vi "TCU Settings Dialog.vi"(8 "error in (no error)":errorcluster, 10 "Message Queues":T11, 11 "TCU Module State Cluster In":T1={"TCU Module Config"={"GUID"="", "Drop Coords"={"Horizontal"=0, "Vertical"=0}, "Process Name"="", "User name"="", "Queue Name"="", "Settings"={"Cycle Period"=500.0, "Setpoint Entry"=0.0, "Output Device"=enum."Default", "Huber Ministat 230 Settings"={"VISA resource name"="", "Simulated?"=TRUE}, "Lauda Settings"={"VISA resource name"="", "Simulated?"=FALSE, "Pump Power"=2}, "Julabo FP-50 Settings"={"VISA resource name"="", "Simulated?"=FALSE, "Pump Power"=2}, "Internal Control?"=FALSE, "Huber Unistat 410 Settings"={"VISA resource name"="", "Address"=0, "Simulated?"=FALSE}}, "Load Count"=0, "Power Level Changed"=FALSE}, "State"=enum."Idle", "Start Time"=timestamp(0 s since 1904-01-01), "Current Time"=timestamp(0 s since 1904-01-01), "First Iteration"=FALSE, "Data"={"TCU Temp"=0.0}, "Process Name"="", "TCU On?"=FALSE, "Power Level Changed"=FALSE} {"TCU Module Config"."Settings"."Huber Unistat 410 Settings"."Address" min=0 max=99 format="%02.0f"; "TCU Module Config"."Settings"."Julabo FP-50 Settings"."Pump Power" min=0 max=8 step=1; "TCU Module Config"."Settings"."Lauda Settings"."Pump Power" min=0 max=8 step=1}) -> (0 "error out":errorcluster, 1 "Cancelled?":bool=TRUE, 2 "UI Refresh Needed?":bool, 3 "TCU Module Config Out":T2={"GUID"="", "Drop Coords"={"Horizontal"=0, "Vertical"=0}, "Process Name"="", "User name"="", "Queue Name"="", "Settings"={"Cycle Period"=0.0, "Setpoint Entry"=0.0, "Output Device"=enum."Default", "Huber Ministat 230 Settings"={"VISA resource name"="", "Simulated?"=FALSE}, "Lauda Settings"={"VISA resource name"="", "Simulated?"=FALSE, "Pump Power"=2}, "Julabo FP-50 Settings"={"VISA resource name"="", "Simulated?"=FALSE, "Pump Power"=2}, "Internal Control?"=FALSE, "Huber Unistat 410 Settings"={"VISA resource name"="", "Address"=0, "Simulated?"=FALSE}}, "Load Count"=0, "Power Level Changed"=FALSE} {"Settings"."Huber Unistat 410 Settings"."Address" min=0 max=99 format="%02.0f"; "Settings"."Julabo FP-50 Settings"."Pump Power" min=0 max=8 step=1; "Settings"."Lauda Settings"."Pump Power" min=0 max=8 step=1})   [LabVIEW 2018, in "TCU Module.lvlib"]
doc: "Dialog for selecting user specified settings."
uses:
  TCU Module.lvlib
  Ismatec ISM 831C/Controls/Ismatech ISM831C Settings Cluster.ctl
  Masterflex 7550-30/Controls/Settings Cluster.ctl
  VICI M50/VICI Settings.ctl
  Measure Instrument/Output Devices.ctl
  Huber TCU/Huber Settings.ctl
  Julabo Type 1 TCU/Julabo Type 1 TCU Folder/Julabo FP-50 Settings.ctl
  Lauda Integral XT-150 TCU/Lauda Settings.ctl
  Huber Unistat 410 TCU/Huber Unistat 410 RS485 Settings.ctl
  All Message Queues.ctl
  support/Message Queue/Message Cluster.ctl
  TCU Module Config Cluster.ctl
  <vilib>/Utility/miscctls.llb/LVPoint32TypeDef.ctl
  TCU Module Settings Cluster.ctl
  TCU Module State Cluster.ctl
  Measure Instrument/State Enum.ctl
  support/Message Queue/Enqueue Message (Single).vi
  <vilib>/Utility/xml.llb/Write to XML File(string).vi
  Settings/Settings.lvlib
  support/Support Library.lvlib
  support/Message Queue/Message Queue.lvlib
  Huber TCU/Huber Ministat 230 TCU.lvlib
  Lauda Integral XT-150 TCU/Lauda TCU.lvlib
  Julabo Type 1 TCU/Julabo Type 1 TCU Folder/Julabo Type FP-50 TCU.lvlib
  Huber Unistat 410 TCU/Huber Unistat 410 TCU.lvlib
  Ismatec ISM 831C/Ismatec ISM 831C.lvlib
  Masterflex 7550-30/Masterflex 7550-30.lvlib
  Measure Instrument/Feed Module Engine.lvlib
panel:
  in  "Module Name":string
  in  "TCU Settings":T15={"TCU Configuration"={"Cycle Period"=500.0, "Ismatech"={"VISA resource name"="", "Simulated?"=FALSE, "Pump Number"=1.0, "Reverse?"=FALSE}, "Masterflex"={"VISA resource name"="", "Simulated?"=FALSE, "Pump Number"=1.0, "Reverse?"=FALSE}, "Setpoint Entry"=0.0, "VICI Settings"={"VISA resource name"="", "Simulated?"=FALSE, "Pump Number"=0.0, "Reverse?"=FALSE}, "Output Device"=enum."Default", "Huber Ministat 230 Settings"={"VISA resource name"="", "Simulated?"=FALSE}, "Julabo Type 1 Settings"={"VISA resource name"="", "Simulated?"=FALSE, "Pump Power"=2}, "Lauda Settings"={"VISA resource name"="", "Simulated?"=FALSE, "Pump Power"=2}, "Control"=enum."Internal", "Huber Unistat 410 Settings"={"VISA resource name"="", "Address"=0, "Simulated?"=FALSE}}, "Stop"=FALSE, "Start"=FALSE} {"TCU Configuration"."Huber Unistat 410 Settings"."Address" min=0 max=99 format="%02.0f"; "TCU Configuration"."Lauda Settings"."Pump Power" min=0 max=8 step=1; "TCU Configuration"."Julabo Type 1 Settings"."Pump Power" min=0 max=8 step=1; "TCU Configuration"."VICI Settings"."Pump Number" min=1.0 max=20.0 step=1.0; "TCU Configuration"."Ismatech"."Pump Number" min=1.0 max=20.0 step=1.0; "TCU Configuration"."Masterflex"."Pump Number" min=1.0 max=20.0 step=1.0}
  in  "Cancel Button":bool
  in  "OK Button":bool
  # "Non visible portion of dialog (needed for connector pane)."
  # "Output Instruments"
  # "Output Instruments"
  # "Output Instruments"
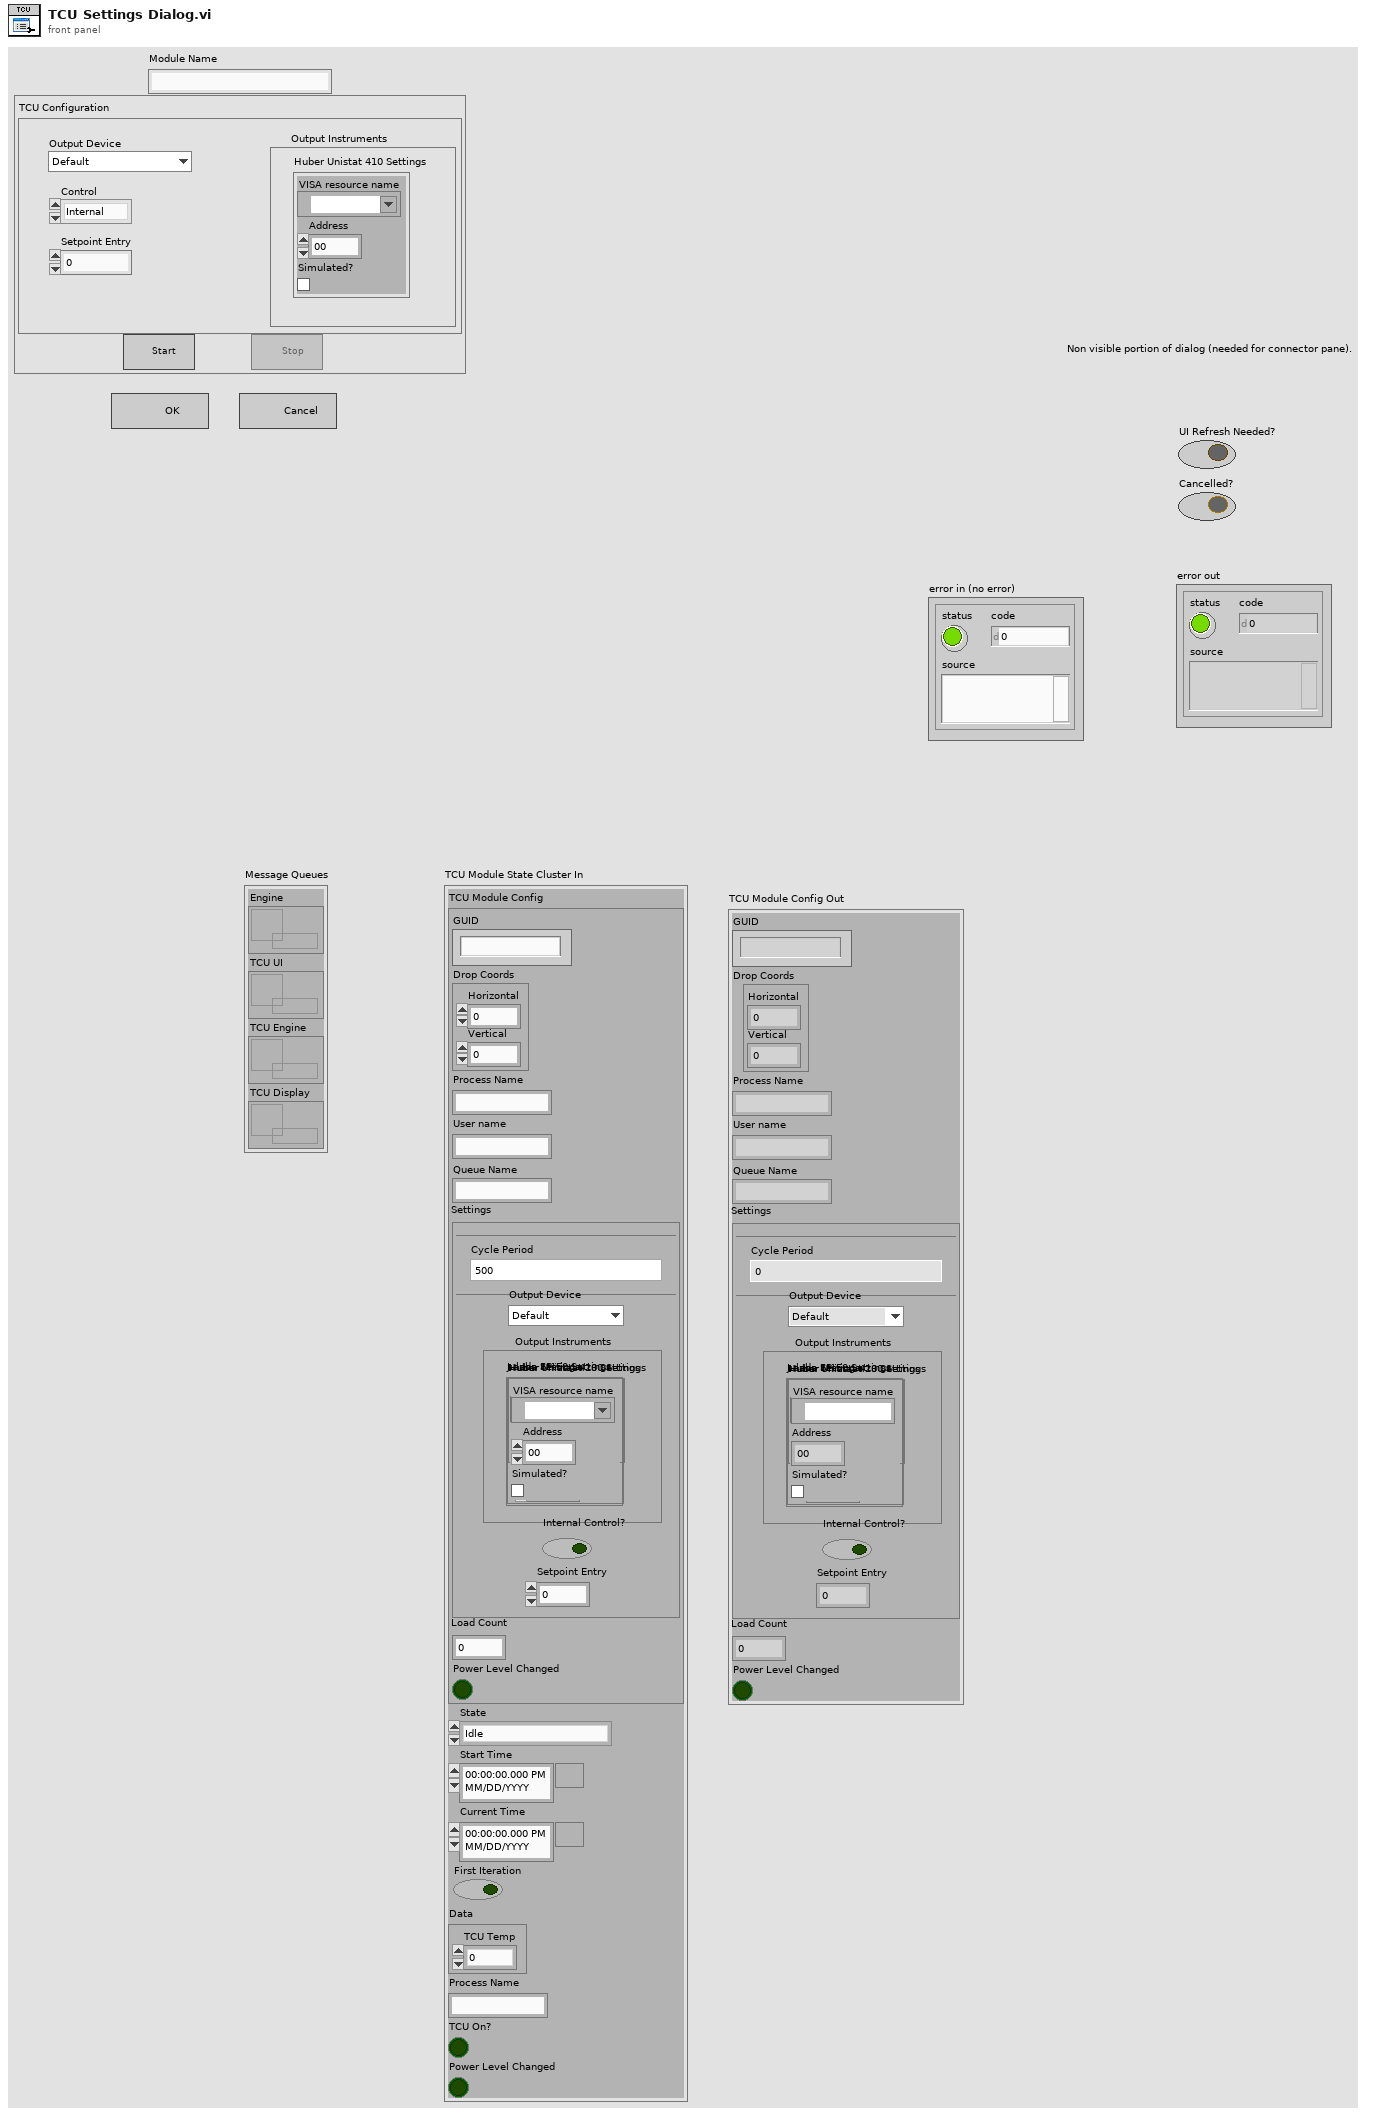
[diagram p1: front panel]
types:
  T1 = typedef "TCU Module.lvlib/TCU Module State Cluster.ctl" = cluster{"TCU Module Config":T2, "State":T10, "Start Time":timestamp, "Current Time":timestamp, "First Iteration":bool, "Data":cluster{"TCU Temp":dbl}, "Process Name":string, "TCU On?":bool, "Power Level Changed":bool}
  T2 = typedef "TCU Module.lvlib/TCU Module Config Cluster.ctl" = cluster{"GUID":string, "Drop Coords":T3, "Process Name":string, "User name":string, "Queue Name":string, "Settings":T4, "Load Count":i32, "Power Level Changed":bool}
  T3 = typedef "LVPoint32TypeDef.ctl" = cluster{"Horizontal":i32, "Vertical":i32}
  T4 = typedef "TCU Module.lvlib/TCU Module Settings Cluster.ctl" = cluster{"Cycle Period":dbl, "Setpoint Entry":dbl, "Output Device":T5, "Huber Ministat 230 Settings":T6, "Lauda Settings":T7, "Julabo FP-50 Settings":T8, "Internal Control?":bool, "Huber Unistat 410 Settings":T9}
  T5 = typedef "Output Devices.ctl" = enum16{"Default", "Huber Ministat 230", "Huber Unistat 410", "Lauda XT-150", "Julabo FP-50"}
  T6 = typedef "Huber Ministat 230 TCU.lvlib/Huber Settings.ctl" = cluster{"VISA resource name":refnum<visa-resource-name>, "Simulated?":bool}
  T7 = typedef "Lauda TCU.lvlib/Lauda Settings.ctl" = cluster{"VISA resource name":refnum<visa-resource-name>, "Simulated?":bool, "Pump Power":i32}
  T8 = typedef "Julabo Type FP-50 TCU.lvlib/Julabo FP-50 Settings.ctl" = cluster{"VISA resource name":refnum<visa-resource-name>, "Simulated?":bool, "Pump Power":i32}
  T9 = typedef "Huber Unistat 410 TCU.lvlib/Huber Unistat 410 RS485 Settings.ctl" = cluster{"VISA resource name":refnum<visa-resource-name>, "Address":i8, "Simulated?":bool}
  T10 = typedef "Feed Module.lvlib/Feed Module Engine.lvlib/State Enum.ctl" = enum16{"Measuring", "Idle", "Paused"}
  T11 = typedef "TCU Module.lvlib/All Message Queues.ctl" = cluster{"Engine":refnum<queue>, "TCU UI":refnum<queue>, "TCU Engine":refnum<queue>, "TCU Display":refnum<queue>}
  T12 = typedef "Ismatec ISM 831C.lvlib/Ismatech ISM831C Settings Cluster.ctl" = cluster{"VISA resource name":refnum<visa-resource-name>, "Simulated?":bool, "Pump Number":dbl, "Reverse?":bool}
  T13 = typedef "Masterflex 7550-30.lvlib/Settings Cluster.ctl" = cluster{"VISA resource name":refnum<visa-resource-name>, "Simulated?":bool, "Pump Number":dbl, "Reverse?":bool}
  T14 = typedef "VICI Settings.ctl" = cluster{"VISA resource name":refnum<visa-resource-name>, "Simulated?":bool, "Pump Number":dbl, "Reverse?":bool}
  T15 = cluster{"TCU Configuration":cluster{"Cycle Period":dbl, "Ismatech":T12, "Masterflex":T13, "Setpoint Entry":dbl, "VICI Settings":T14, "Output Device":T5, "Huber Ministat 230 Settings":T6, "Julabo Type 1 Settings":T8, "Lauda Settings":T7, "Control":enum16{"Internal", "External"}, "Huber Unistat 410 Settings":T9}, "Stop":bool, "Start":bool}
  T16 = enum8{"Enabled", "Disabled", "Disabled and Grayed Out"}
  T17 = typedef "Ismatec ISM 831C.lvlib/Ismatech Settings Cluster.ctl" = cluster{"VISA resource name":refnum<visa-resource-name>, "Simulated?":bool, "Pump Number":dbl, "Reverse?":bool}
  T18 = cluster{"Cycle Period":dbl, "Ismatech":T17, "Masterflex":T13, "Setpoint Entry":dbl, "VICI Settings":T14, "Output Device":T5, "Huber Ministat 230 Settings":T6, "Julabo Type 1 Settings":T8, "Lauda Settings":T7, "Control":enum16{"Internal", "External"}, "Huber Unistat 410 Settings":T9}
  T19 = cluster{"Cycle Period":dbl, "Ismatech":T12, "Masterflex":T13, "Setpoint Entry":dbl, "VICI Settings":T14, "Output Device":T5, "Huber Ministat 230 Settings":T6, "Julabo Type 1 Settings":T8, "Lauda Settings":T7, "Control":enum16{"Internal", "External"}, "Huber Unistat 410 Settings":T9}
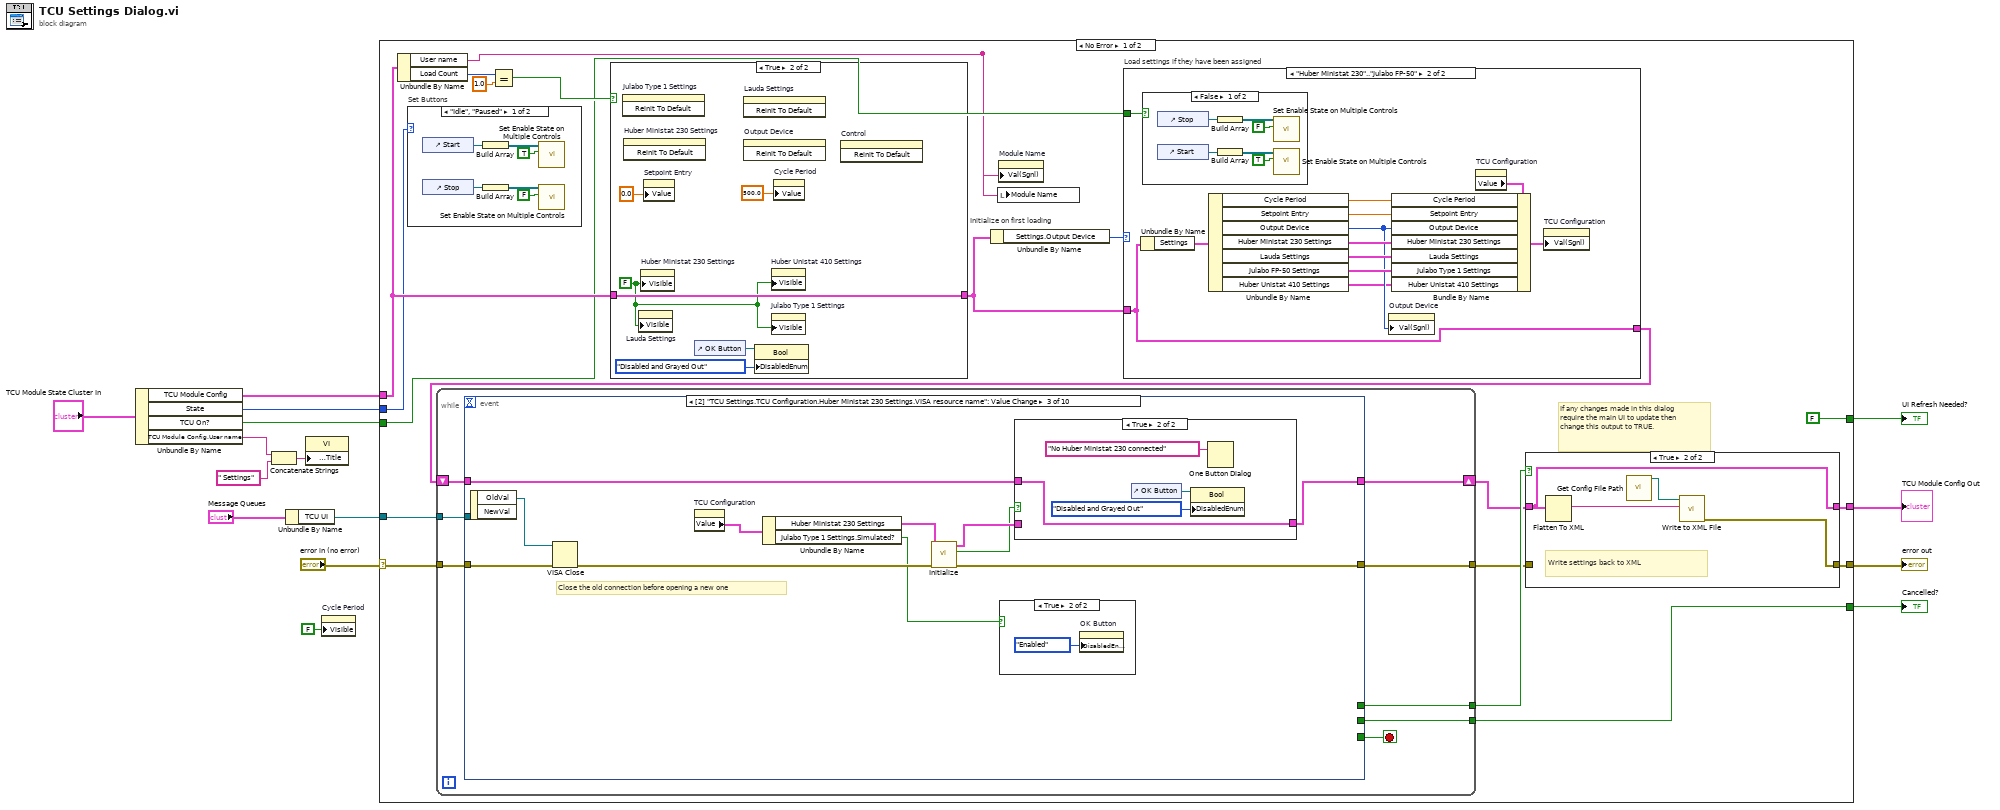
[diagram p0: block diagram]
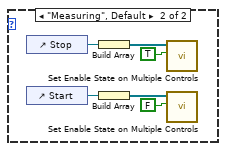
[diagram p2: hidden frame]
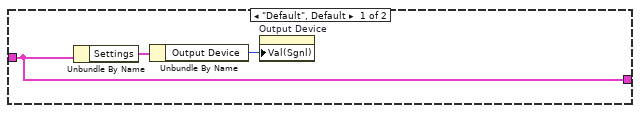
[diagram p3: hidden frame]
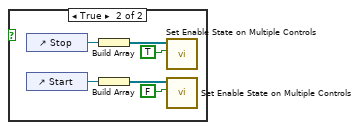
[diagram p4: hidden frame]
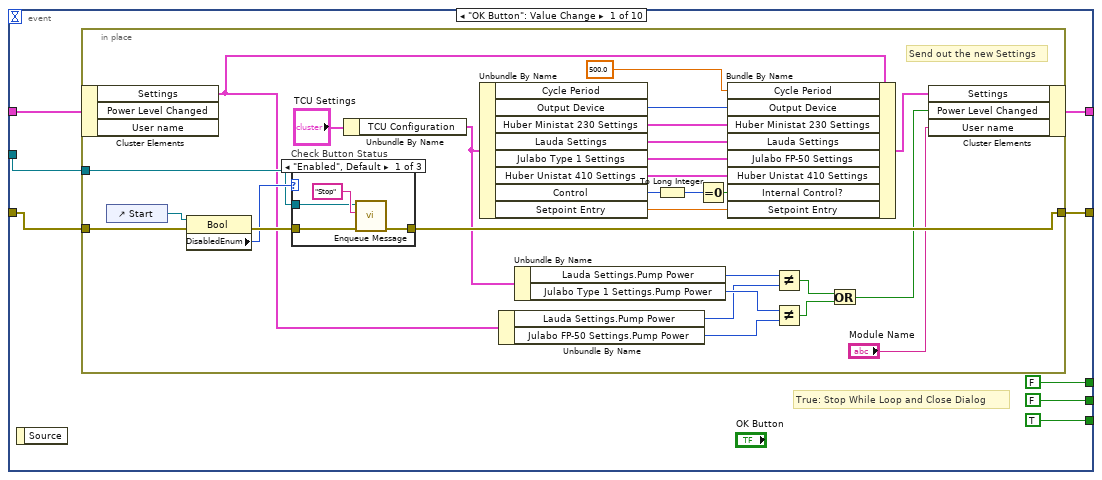
[diagram p6: hidden frame]
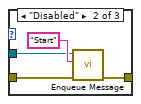
[diagram p7: hidden frame]
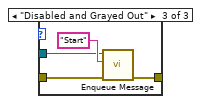
[diagram p8: hidden frame]
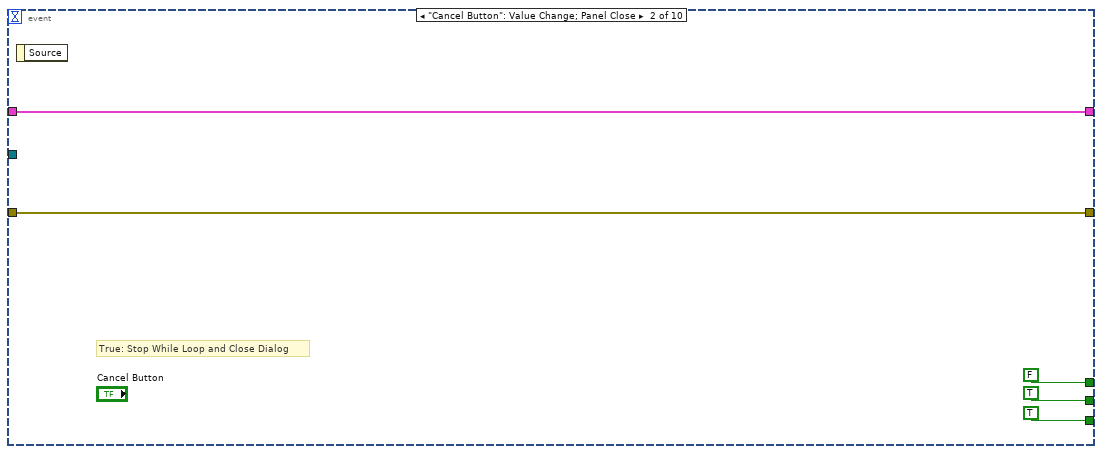
[diagram p9: hidden frame]
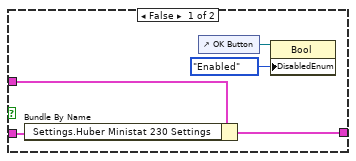
[diagram p11: hidden frame]
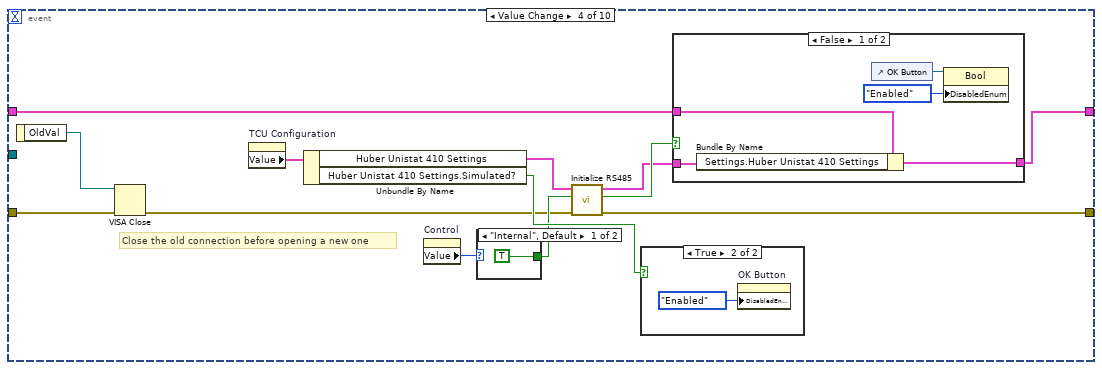
[diagram p12: hidden frame]
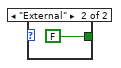
[diagram p14: hidden frame]
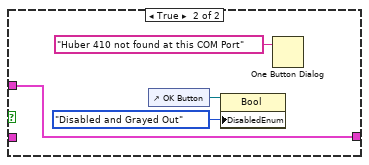
[diagram p15: hidden frame]
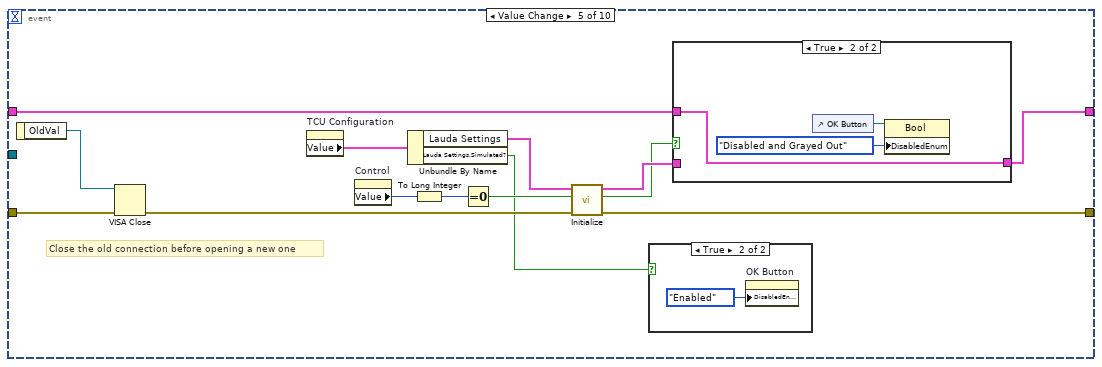
[diagram p16: hidden frame]
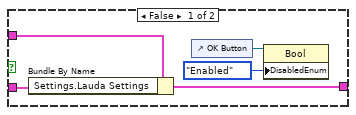
[diagram p18: hidden frame]
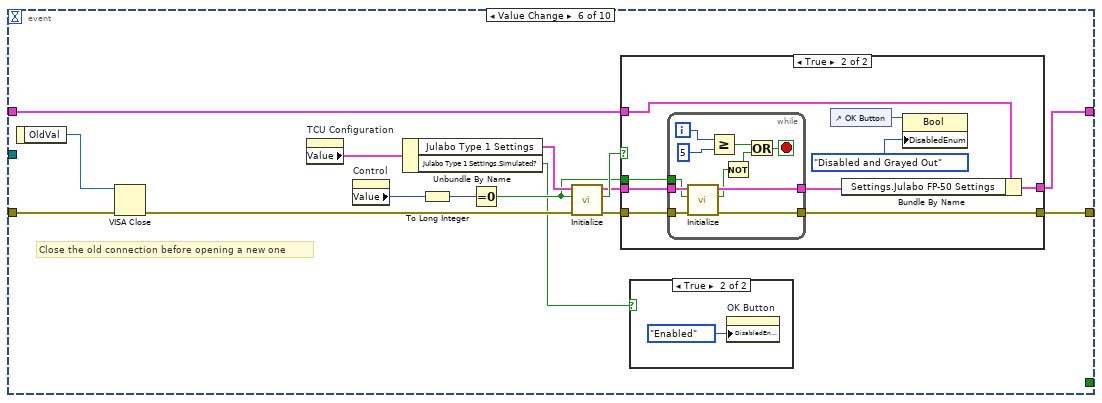
[diagram p19: hidden frame]
diagram:
  n1 = Unbundle By Name("TCU Module State Cluster In") -> ("TCU Module Config"=w7:T2, "State"=w6:T10, "TCU On?"=w4:bool, "TCU Module Config.User name"=w1:string)
  n2 = Concatenate Strings(w1, " Settings" ("string")) -> (w3:string)
  n3 = Unbundle By Name("Message Queues") -> ("TCU UI"=w12:refnum<queue>)
  n4 = property class="VI"("Front Panel.Title"=w3) -> ()  [unwired: 2 in, 2 out]
  n5 = property on="Cycle Period" class="DigNum (strict)"("Visible"=FALSE) -> ()  [unwired: 2 in, 2 out]
  n6 = case shown="No Error" "error in (no error)" {
    selector: "error in (no error)" -> [w21 w309]
    tunnel: [w24 w309] -> w15
    tunnel: w7 -> [w20 w307]
    tunnel: [w28 w307] -> w9
    tunnel: [FALSE ("UI Refresh Needed?") _] -> w14
    tunnel: [w31 TRUE ("UI Refresh Needed?")] -> w13
    tunnel: w12 -> [w22 _]
    tunnel: w6 -> [w18 _]
    tunnel: w4 -> [w17 _]
    frame No Error {
      # "If any changes made in this dialog require the main UI to update then change this output to TRUE."
      n7 = Unbundle By Name(w20) -> ("User name"=w16:string, "Load Count"=w33:i32)
      n8 = case "Set Buttons" shown="\"Idle\", \"Paused\"" w18 {
        frame "Idle", "Paused" {
          n9 = control-ref of="Start"() -> (w35:refnum<vi>)
          n10 = control-ref of="Stop"() -> (w37:refnum<vi>)
          n11 = Build Array(w35) -> (w39:refnum<vi>[])
          n12 = Build Array(w37) -> (w36:refnum<vi>[])
          n13 = call "Set Enable State on Multiple Controls.vi"("Enable?"=TRUE, "Controls"=w39) -> ()  [unwired: 10 in]
          n14 = call "Set Enable State on Multiple Controls.vi"("Enable?"=FALSE, "Controls"=w36) -> ()  [unwired: 10 in]
        }
        frame "Measuring", Default {
          n15 = control-ref of="Stop"() -> (w41:refnum<vi>)
          n16 = control-ref of="Start"() -> (w42:refnum<vi>)
          n17 = Build Array(w41) -> (w45:refnum<vi>[])
          n18 = Build Array(w42) -> (w43:refnum<vi>[])
          n19 = call "Set Enable State on Multiple Controls.vi"("Enable?"=TRUE, "Controls"=w45) -> ()  [unwired: 10 in]
          n20 = call "Set Enable State on Multiple Controls.vi"("Enable?"=FALSE, "Controls"=w43) -> ()  [unwired: 10 in]
        }
      }
      n21 = Equal?(x=w33, y=1.0) -> (x = y?=w27:bool)
      n22 = case "Initialize on first loading" shown="True" w27 {
        tunnel: w20 -> [w74 w80]
        tunnel: [w74 w80] -> w29
        frame False {
        }
        frame True {
          w75 = FALSE ("Visible")
          n23 = invoke on="Julabo Type 1 Settings" class="Clust (strict)" method="Reinit To Default"() -> ()  [unwired: 3 in, 3 out]
          n24 = invoke on="Huber Ministat 230 Settings" class="Clust (strict)" method="Reinit To Default"() -> ()  [unwired: 3 in, 3 out]
          n25 = property on="Lauda Settings" class="Clust (strict)"("Visible"=w75) -> ()  [unwired: 2 in, 2 out]
          n26 = property on="Huber Ministat 230 Settings" class="Clust (strict)"("Visible"=w75) -> ()  [unwired: 2 in, 2 out]
          n27 = property on="Setpoint Entry" class="DigNum (strict)"("Value"=0.0) -> ()  [unwired: 2 in, 2 out]
          n28 = control-ref of="OK Button"() -> (w77:refnum<vi>)
          n29 = invoke on="Lauda Settings" class="Clust (strict)" method="Reinit To Default"() -> ()  [unwired: 3 in, 3 out]
          n30 = invoke on="Output Device" class="Enum (strict)" method="Reinit To Default"() -> ()  [unwired: 3 in, 3 out]
          n31 = property class="Bool"(reference=w77, "DisabledEnum"=T16."Disabled and Grayed Out" ("Disabled")) -> ()  [unwired: 1 in, 2 out]
          n32 = property on="Huber Unistat 410 Settings" class="Clust (strict)"("Visible"=w75) -> ()  [unwired: 2 in, 2 out]
          n33 = property on="Julabo Type 1 Settings" class="Clust (strict)"("Visible"=w75) -> ()  [unwired: 2 in, 2 out]
          n34 = property on="Cycle Period" class="DigNum (strict)"("Value"=500.0) -> ()  [unwired: 2 in, 2 out]
          n35 = invoke on="Control" class="Enum (strict)" method="Reinit To Default"() -> ()  [unwired: 3 in, 3 out]
        }
      }
      n36 = Unbundle By Name(w29) -> ("Settings.Output Device"=w30:T5)
      n37 = local write "Module Name"(w16) -> ()
      n38 = property on="Module Name" class="Str"("Val(Sgnl)"=w16) -> ()  [unwired: 2 in, 2 out]
      n39 = case "Load settings if they have been assigned" shown="\"Huber Ministat 230\"..\"Julabo FP-50\"" w30 {
        tunnel: w29 -> [w47 w51]
        tunnel: [w47 w51] -> w19
        tunnel: w17 -> [_ w54]
        frame "Default", Default {
          n40 = Unbundle By Name(w47) -> ("Settings"=w49:T4)
          n41 = Unbundle By Name(w49) -> ("Output Device"=w48:T5)
          n42 = property on="Output Device" class="Enum (strict)"("Val(Sgnl)"=w48) -> ()  [unwired: 2 in, 2 out]
        }
        frame "Huber Ministat 230".."Julabo FP-50" {
          n43 = Unbundle By Name(w51) -> ("Settings"=w59:T4)
          n44 = case shown="False" w54 {
            frame False {
              n45 = control-ref of="Stop"() -> (w64:refnum<vi>)
              n46 = control-ref of="Start"() -> (w65:refnum<vi>)
              n47 = Build Array(w64) -> (w66:refnum<vi>[])
              n48 = Build Array(w65) -> (w67:refnum<vi>[])
              n49 = call "Set Enable State on Multiple Controls.vi"("Enable?"=FALSE, "Controls"=w66) -> ()  [unwired: 10 in]
              n50 = call "Set Enable State on Multiple Controls.vi"("Enable?"=TRUE, "Controls"=w67) -> ()  [unwired: 10 in]
            }
            frame True {
              n51 = control-ref of="Stop"() -> (w70:refnum<vi>)
              n52 = control-ref of="Start"() -> (w71:refnum<vi>)
              n53 = Build Array(w70) -> (w72:refnum<vi>[])
              n54 = Build Array(w71) -> (w73:refnum<vi>[])
              n55 = call "Set Enable State on Multiple Controls.vi"("Enable?"=TRUE, "Controls"=w72) -> ()  [unwired: 10 in]
              n56 = call "Set Enable State on Multiple Controls.vi"("Enable?"=FALSE, "Controls"=w73) -> ()  [unwired: 10 in]
            }
          }
          n57 = Unbundle By Name(w59) -> ("Cycle Period"=w61:dbl, "Setpoint Entry"=w57:dbl, "Output Device"=w52:T5, "Huber Ministat 230 Settings"=w58:T6, "Lauda Settings"=w56:T7, "Julabo FP-50 Settings"=w55:T8, "Huber Unistat 410 Settings"=w50:T9)
          n58 = property on="Output Device" class="Enum (strict)"("Val(Sgnl)"=w52) -> ()  [unwired: 2 in, 2 out]
          n59 = property on="TCU Configuration" class="Clust (strict)"() -> ("Value"=w53:T18)  [unwired: 2 in, 2 out]
          n60 = Bundle By Name(cluster=w53, "Cycle Period"=w61, "Setpoint Entry"=w57, "Output Device"=w52, "Huber Ministat 230 Settings"=w58, "Lauda Settings"=w56, "Julabo Type 1 Settings"=w55, "Huber Unistat 410 Settings"=w50) -> (w60:T18)
          n61 = property on="TCU Configuration" class="Clust (strict)"("Val(Sgnl)"=w60) -> ()  [unwired: 2 in, 2 out]
        }
      }
      n62 = while {
        tunnel: [w88] -> w26
        tunnel: [w86] -> w31
        tunnel: [w84] -> w23
        tunnel: w22 -> [w83]
        tunnel: w21 -> [w82]
        shift-right: [w85] -> w25
        shift-left: w19 -> [w81]
        stop <- w87 stop-if-true
        n63 = event shown="[2] \"TCU Settings.TCU Configuration.Huber Ministat 230 Settings.VISA resource name\": Value Change" {
          selector: _ -> [_ _ _ _ _ _ _ _ _ _]
          dyn-events: _ -> [_ _ _ _ _ _ _ _ _ _]
          timeout: _ -> [_ _ _ _ _ _ _ _ _ _]
          tunnel: [FALSE ("UI Refresh Needed?") FALSE ("UI Refresh Needed?") _ _ _ _ _ _ _ _] -> w88
          tunnel: [TRUE TRUE _ _ _ _ _ _ _ _] -> w87
          tunnel: [FALSE ("UI Refresh Needed?") TRUE ("UI Refresh Needed?") _ _ _ _ _ _ _ _] -> w86
          tunnel: w81 -> [w90 w138 w150 w173 w199 w216 w254 w281 w286 w294]
          tunnel: [w89 w138 w149 w172 w198 w215 w253 w281 w286 w294] -> w85
          tunnel: [w93 w137 w146 w163 w193 w213 _ _ w285 w293] -> w84
          tunnel: w83 -> [w92 _ _ _ _ _ _ _ _ _]
          tunnel: w82 -> [w91 w137 w148 w171 w197 w223 _ _ w285 w293]
          event "OK Button": Value Change {
            # "True: Stop While Loop and Close Dialog"
            n64 = event-data() -> ()  [unwired: 1 in, 1 out]
            n65 = in-place {
              in-place-border: [w120] -> w93
              in-place-border: w92 -> [w119]
              in-place-border: w91 -> [w118]
              # "Send out the new Settings"
              n66 = in-place-cluster #1(w90) -> ("Settings"=w98:T4)  [unwired: 2 out]
              n67 = control-ref of="Start"() -> (w123:refnum<vi>)
              n68 = property class="Bool"(reference=w123, error in=w118) -> (error out=w124:errorcluster, "DisabledEnum"=w121:T16)  [unwired: 1 out]
              n69 = case "Check Button Status" shown="\"Enabled\", Default" w121 {
                tunnel: w124 -> [w126 w131 w135]
                tunnel: [w128 w130 w134] -> w120
                tunnel: w119 -> [w125 w129 w133]
                frame "Enabled", Default {
                  n70 = call-poly "Enqueue Message.vi"("error in (no error)"=w126, "Message"="Stop", "Message Queue"=w125) -> ("error out"=w128:errorcluster)  [unwired: 7 in, 1 out]
                }
                frame "Disabled" {
                  n71 = call-poly "Enqueue Message.vi"("error in (no error)"=w131, "Message"="Start", "Message Queue"=w129) -> ("error out"=w130:errorcluster)  [unwired: 7 in, 1 out]
                }
                frame "Disabled and Grayed Out" {
                  n72 = call-poly "Enqueue Message.vi"("error in (no error)"=w135, "Message"="Start", "Message Queue"=w133) -> ("error out"=w134:errorcluster)  [unwired: 7 in, 1 out]
                }
              }
              n73 = Unbundle By Name("TCU Settings") -> ("TCU Configuration"=w108:T19)
              n74 = Unbundle By Name(w108) -> ("Output Device"=w117:T5, "Huber Ministat 230 Settings"=w112:T6, "Lauda Settings"=w113:T7, "Julabo Type 1 Settings"=w116:T8, "Huber Unistat 410 Settings"=w97:T9, "Control"=w111:enum16{"Internal", "External"}, "Setpoint Entry"=w114:dbl)  [unwired: 1 out]
              n75 = Unbundle By Name(w98) -> ("Lauda Settings.Pump Power"=w100:i32, "Julabo FP-50 Settings.Pump Power"=w99:i32)
              n76 = Unbundle By Name(w108) -> ("Lauda Settings.Pump Power"=w107:i32, "Julabo Type 1 Settings.Pump Power"=w104:i32)
              n77 = To Long Integer(number=w111) -> (32bit integer=w110:i32)
              n78 = Equal To 0?(x=w110) -> (x = 0?=w109:bool)
              n79 = Bundle By Name(cluster=w98, "Cycle Period"=500.0, "Output Device"=w117, "Huber Ministat 230 Settings"=w112, "Lauda Settings"=w113, "Julabo FP-50 Settings"=w116, "Huber Unistat 410 Settings"=w97, "Internal Control?"=w109, "Setpoint Entry"=w114) -> (w103:T4)
              n80 = Not Equal?(x=w107, y=w100) -> (x != y?=w106:bool)
              n81 = Not Equal?(x=w104, y=w99) -> (x != y?=w105:bool)
              n82 = Or(x=w106, y=w105) -> (x .or. y?=w102:bool)
              n83 = in-place-cluster #1("Settings"=w103, "Power Level Changed"=w102, "User name"="Module Name") -> (w89:T2)
            }
          }
          event "Cancel Button": Value Change; Panel Close {
            # "True: Stop While Loop and Close Dialog"
            n84 = event-data() -> ()  [unwired: 1 in, 1 out]
          }
          event Value Change {
            # "Close the old connection before opening a new one"
            n85 = event-data() -> ("OldVal"=w151:refnum<visa-resource-name>)  [unwired: 1 in, 1 out]
            n86 = VISA Close(VISA resource name=w151, error in (no error)=w148) -> (error out=w147:errorcluster)
            n87 = property on="TCU Configuration" class="Clust (strict)"() -> ("Value"=w152:T18)  [unwired: 2 in, 2 out]
            n88 = Unbundle By Name(w152) -> ("Huber Ministat 230 Settings"=w145:T6, "Julabo Type 1 Settings.Simulated?"=w142:bool)
            n89 = call "Initialize.vi"("error in (no error)"=w147, "Huber Settings"=w145) -> ("error out"=w146:errorcluster, "Connection Error"=w143:bool, "Huber Settings"=w144:T6)  [unwired: 7 in]
            n90 = case shown="True" w142 {
              frame False {
              }
              frame True {
                n91 = property on="OK Button" class="Bool"("DisabledEnum"=T16."Enabled" ("Disabled")) -> ()  [unwired: 2 in, 2 out]
              }
            }
            n92 = case shown="True" w143 {
              tunnel: w144 -> [w158 _]
              tunnel: w150 -> [w154 w162]
              tunnel: [w157 w162] -> w149
              frame False {
                n93 = Bundle By Name(cluster=w154, "Settings.Huber Ministat 230 Settings"=w158) -> (w157:T2)
                n94 = control-ref of="OK Button"() -> (w155:refnum<vi>)
                n95 = property class="Bool"(reference=w155, "DisabledEnum"=T16."Enabled" ("Disabled")) -> ()  [unwired: 1 in, 2 out]
              }
              frame True {
                n96 = control-ref of="OK Button"() -> (w160:refnum<vi>)
                n97 = property class="Bool"(reference=w160, "DisabledEnum"=T16."Disabled and Grayed Out" ("Disabled")) -> ()  [unwired: 1 in, 2 out]
                n98 = One Button Dialog(message="No Huber Ministat 230 connected") -> ()  [unwired: 1 in, 1 out]
              }
            }
          }
          event Value Change {
            # "Close the old connection before opening a new one"
            n99 = event-data() -> ("OldVal"=w174:refnum<visa-resource-name>)  [unwired: 1 in]
            n100 = VISA Close(VISA resource name=w174, error in (no error)=w171) -> (error out=w166:errorcluster)
            n101 = property on="TCU Configuration" class="Clust (strict)"() -> ("Value"=w175:T18)  [unwired: 2 in, 2 out]
            n102 = Unbundle By Name(w175) -> ("Huber Unistat 410 Settings"=w168:T9, "Huber Unistat 410 Settings.Simulated?"=w169:bool)
            n103 = property on="Control" class="Enum (strict)"() -> ("Value"=w170:enum16{"Internal", "External"})  [unwired: 2 in, 2 out]
            n104 = case shown="\"Internal\", Default" w170 {
              tunnel: [TRUE FALSE] -> w167
              frame "Internal", Default {
              }
              frame "External" {
              }
            }
            n105 = call "Initialize RS485.vi"("error in (no error)"=w166, "Internal?"=w167, "Huber Unistat 410 Settings"=w168) -> ("error out"=w163:errorcluster, "Connection Error"=w165:bool, "Huber Unistat 410 Settings 2"=w164:T9)  [unwired: 6 in]
            n106 = case shown="True" w169 {
              frame False {
              }
              frame True {
                n107 = property on="OK Button" class="Bool"("DisabledEnum"=T16."Enabled" ("Disabled")) -> ()  [unwired: 2 in, 2 out]
              }
            }
            n108 = case shown="False" w165 {
              tunnel: w164 -> [w183 _]
              tunnel: w173 -> [w179 w187]
              tunnel: [w182 w187] -> w172
              frame False {
                n109 = Bundle By Name(cluster=w179, "Settings.Huber Unistat 410 Settings"=w183) -> (w182:T2)
                n110 = control-ref of="OK Button"() -> (w180:refnum<vi>)
                n111 = property class="Bool"(reference=w180, "DisabledEnum"=T16."Enabled" ("Disabled")) -> ()  [unwired: 1 in, 2 out]
              }
              frame True {
                n112 = control-ref of="OK Button"() -> (w185:refnum<vi>)
                n113 = property class="Bool"(reference=w185, "DisabledEnum"=T16."Disabled and Grayed Out" ("Disabled")) -> ()  [unwired: 1 in, 2 out]
                n114 = One Button Dialog(message="Huber 410 not found at this COM Port") -> ()  [unwired: 1 in, 1 out]
              }
            }
          }
          event Value Change {
            # "Close the old connection before opening a new one"
            n115 = event-data() -> ("OldVal"=w200:refnum<visa-resource-name>)  [unwired: 1 in]
            n116 = VISA Close(VISA resource name=w200, error in (no error)=w197) -> (error out=w196:errorcluster)
            n117 = property on="TCU Configuration" class="Clust (strict)"() -> ("Value"=w201:T18)  [unwired: 2 in, 2 out]
            n118 = property on="Control" class="Enum (strict)"() -> ("Value"=w189:enum16{"Internal", "External"})  [unwired: 2 in, 2 out]
            n119 = Unbundle By Name(w201) -> ("Lauda Settings"=w195:T7, "Lauda Settings.Simulated?"=w188:bool)
            n120 = To Long Integer(number=w189) -> (32bit integer=w190:i32)
            n121 = Equal To 0?(x=w190) -> (x = 0?=w192:bool)
            n122 = call "Initialize.vi"("error in (no error)"=w196, "Internal?"=w192, "Lauda Settings In"=w195) -> ("error out"=w193:errorcluster, "Connection Error"=w191:bool, "Lauda Settings Out"=w194:T7)  [unwired: 6 in]
            n123 = case shown="True" w188 {
              frame False {
              }
              frame True {
                n124 = property on="OK Button" class="Bool"("DisabledEnum"=T16."Enabled" ("Disabled")) -> ()  [unwired: 2 in, 2 out]
              }
            }
            n125 = case shown="True" w191 {
              tunnel: w194 -> [w207 _]
              tunnel: w199 -> [w203 w210]
              tunnel: [w206 w210] -> w198
              frame False {
                n126 = Bundle By Name(cluster=w203, "Settings.Lauda Settings"=w207) -> (w206:T2)
                n127 = control-ref of="OK Button"() -> (w204:refnum<vi>)
                n128 = property class="Bool"(reference=w204, "DisabledEnum"=T16."Enabled" ("Disabled")) -> ()  [unwired: 1 in, 2 out]
              }
              frame True {
                n129 = control-ref of="OK Button"() -> (w208:refnum<vi>)
                n130 = property class="Bool"(reference=w208, "DisabledEnum"=T16."Disabled and Grayed Out" ("Disabled")) -> ()  [unwired: 1 in, 2 out]
              }
            }
          }
          event Value Change {
            # "Close the old connection before opening a new one"
            n131 = event-data() -> ("OldVal"=w224:refnum<visa-resource-name>)  [unwired: 1 in]
            n132 = VISA Close(VISA resource name=w224, error in (no error)=w223) -> (error out=w222:errorcluster)
            n133 = property on="TCU Configuration" class="Clust (strict)"() -> ("Value"=w225:T18)  [unwired: 2 in, 2 out]
            n134 = property on="Control" class="Enum (strict)"() -> ("Value"=w219:enum16{"Internal", "External"})  [unwired: 2 in, 2 out]
            n135 = Unbundle By Name(w225) -> ("Julabo Type 1 Settings"=w221:T8, "Julabo Type 1 Settings.Simulated?"=w211:bool)
            n136 = To Long Integer(number=w219) -> (32bit integer=w220:i32)
            n137 = Equal To 0?(x=w220) -> (x = 0?=w212:bool)
            n138 = call "Initialize.vi"("error in (no error)"=w222, "Internal?"=w212, "Julabo FP-50 Settings"=w221) -> ("error out"=w214:errorcluster, "Connection Error"=w218:bool, "Julabo FP-50 Settings"=w217:T8)  [unwired: 6 in]
            n139 = case shown="True" w218 {
              tunnel: w217 -> [w230 w241]
              tunnel: w216 -> [w229 w238]
              tunnel: [w228 w239] -> w215
              tunnel: w214 -> [w227 w235]
              tunnel: [w227 w234] -> w213
              tunnel: w212 -> [_ w233]
              frame False {
                n140 = Bundle By Name(cluster=w229, "Settings.Julabo FP-50 Settings"=w230) -> (w228:T2)
                n141 = control-ref of="OK Button"() -> (w232:refnum<vi>)
                n142 = property class="Bool"(reference=w232, "DisabledEnum"=T16."Enabled" ("Disabled")) -> ()  [unwired: 1 in, 2 out]
              }
              frame True {
                n143 = while {
                  tunnel: w241 -> [w252]
                  tunnel: [w251] -> w240
                  tunnel: w235 -> [w246]
                  tunnel: [w245] -> w234
                  tunnel: w233 -> [w242]
                  i -> [w249]
                  stop <- w247 stop-if-true
                  n144 = call "Initialize.vi"("error in (no error)"=w246, "Internal?"=w242, "Julabo FP-50 Settings"=w252) -> ("error out"=w245:errorcluster, "Connection Error"=w250:bool, "Julabo FP-50 Settings"=w251:T8)  [unwired: 6 in]
                  n145 = Greater Or Equal?(x=w249, y=5) -> (x >= y?=w243:bool)
                  n146 = Not(x=w250) -> (.not. x?=w244:bool)
                  n147 = Or(x=w243, y=w244) -> (x .or. y?=w247:bool)
                }
                n148 = control-ref of="OK Button"() -> (w237:refnum<vi>)
                n149 = Bundle By Name(cluster=w238, "Settings.Julabo FP-50 Settings"=w240) -> (w239:T2)
                n150 = property class="Bool"(reference=w237, "DisabledEnum"=T16."Disabled and Grayed Out" ("Disabled")) -> ()  [unwired: 1 in, 2 out]
              }
            }
            n151 = case shown="True" w211 {
              frame False {
              }
              frame True {
                n152 = property on="OK Button" class="Bool"("DisabledEnum"=T16."Enabled" ("Disabled")) -> ()  [unwired: 2 in, 2 out]
              }
            }
          }
          event Value Change {
            n153 = event-data() -> ("NewVal"=w255:T5)  [unwired: 1 in]
            n154 = case "Selected Device" shown="\"Huber Unistat 410\"" w255 {
              tunnel: w254 -> [w260 w265 w266 w272 w277]
              tunnel: [w260 w265 w266 w272 w277] -> w253
              frame "Default", Default {
                n155 = property on="Huber Unistat 410 Settings" class="Clust (strict)"("Visible"=FALSE) -> ()  [unwired: 2 in, 2 out]
                n156 = property on="Julabo Type 1 Settings" class="Clust (strict)"("Visible"=FALSE) -> ()  [unwired: 2 in, 2 out]
                n157 = property on="Lauda Settings" class="Clust (strict)"("Visible"=FALSE) -> ()  [unwired: 2 in, 2 out]
                n158 = property on="Huber Ministat 230 Settings" class="Clust (strict)"("Visible"=FALSE) -> ()  [unwired: 2 in, 2 out]
              }
              frame "Huber Ministat 230" {
                n159 = property on="Huber Unistat 410 Settings" class="Clust (strict)"("Visible"=FALSE) -> ()  [unwired: 2 in, 2 out]
                n160 = property on="Julabo Type 1 Settings" class="Clust (strict)"("Visible"=FALSE) -> ()  [unwired: 2 in, 2 out]
                n161 = property on="Lauda Settings" class="Clust (strict)"("Visible"=FALSE) -> ()  [unwired: 2 in, 2 out]
                n162 = property on="Huber Ministat 230 Settings" class="Clust (strict)"("Visible"=TRUE) -> ()  [unwired: 2 in, 2 out]
              }
              frame "Huber Unistat 410" {
                n163 = property on="Huber Unistat 410 Settings" class="Clust (strict)"("Visible"=TRUE) -> ()  [unwired: 2 in, 2 out]
                n164 = property on="Julabo Type 1 Settings" class="Clust (strict)"("Visible"=FALSE) -> ()  [unwired: 2 in, 2 out]
                n165 = property on="Lauda Settings" class="Clust (strict)"("Visible"=FALSE) -> ()  [unwired: 2 in, 2 out]
                n166 = property on="Huber Ministat 230 Settings" class="Clust (strict)"("Visible"=FALSE) -> ()  [unwired: 2 in, 2 out]
              }
              frame "Lauda XT-150" {
                n167 = property on="Huber Unistat 410 Settings" class="Clust (strict)"("Visible"=FALSE) -> ()  [unwired: 2 in, 2 out]
                n168 = property on="Julabo Type 1 Settings" class="Clust (strict)"("Visible"=FALSE) -> ()  [unwired: 2 in, 2 out]
                n169 = property on="Lauda Settings" class="Clust (strict)"("Visible"=TRUE) -> ()  [unwired: 2 in, 2 out]
                n170 = property on="Huber Ministat 230 Settings" class="Clust (strict)"("Visible"=FALSE) -> ()  [unwired: 2 in, 2 out]
              }
              frame "Julabo FP-50" {
                n171 = property on="Huber Unistat 410 Settings" class="Clust (strict)"("Visible"=FALSE) -> ()  [unwired: 2 in, 2 out]
                n172 = property on="Julabo Type 1 Settings" class="Clust (strict)"("Visible"=TRUE) -> ()  [unwired: 2 in, 2 out]
                n173 = property on="Lauda Settings" class="Clust (strict)"("Visible"=FALSE) -> ()  [unwired: 2 in, 2 out]
                n174 = property on="Huber Ministat 230 Settings" class="Clust (strict)"("Visible"=FALSE) -> ()  [unwired: 2 in, 2 out]
              }
            }
          }
          event Value Change {
            n175 = event-data() -> ("NewVal"=w282:bool)  [unwired: 1 in]
            n176 = case shown="True" w282 {
              frame False {
                n177 = property on="OK Button" class="Bool"("DisabledEnum"=T16."Disabled and Grayed Out" ("Disabled")) -> ()  [unwired: 2 in, 2 out]
              }
              frame True {
                n178 = property on="OK Button" class="Bool"("DisabledEnum"=T16."Enabled" ("Disabled")) -> ()  [unwired: 2 in, 2 out]
              }
            }
          }
          event "TCU Settings.Start": Value Change {
            # "Enable Stop"
            # "Disable and Gray out Start"
            n179 = event-data() -> ()  [unwired: 1 in, 6 out]
            n180 = control-ref of="Start"() -> (w288:refnum<vi>)
            n181 = control-ref of="Stop"() -> (w287:refnum<vi>)
            n182 = Build Array(w288) -> (w290:refnum<vi>[])
            n183 = Build Array(w287) -> (w292:refnum<vi>[])
            n184 = call "Set Enable State on Multiple Controls.vi"("Enable?"=FALSE, "Controls"=w290) -> ()  [unwired: 10 in]
            n185 = call "Set Enable State on Multiple Controls.vi"("Enable?"=TRUE, "Controls"=w292) -> ()  [unwired: 10 in]
          }
          event "TCU Settings.Stop": Value Change {
            # "Enable Start"
            # "Disable and Gray out Stop"
            n186 = event-data() -> ()  [unwired: 1 in, 1 out]
            n187 = control-ref of="Stop"() -> (w295:refnum<vi>)
            n188 = control-ref of="Start"() -> (w296:refnum<vi>)
            n189 = Build Array(w295) -> (w298:refnum<vi>[])
            n190 = Build Array(w296) -> (w300:refnum<vi>[])
            n191 = call "Set Enable State on Multiple Controls.vi"("Enable?"=FALSE, "Controls"=w298) -> ()  [unwired: 10 in]
            n192 = call "Set Enable State on Multiple Controls.vi"("Enable?"=TRUE, "Controls"=w300) -> ()  [unwired: 10 in]
          }
        }
      }
      n193 = case shown="True" w26 {
        tunnel: w25 -> [w302 w303]
        tunnel: [w301 w304] -> w24
        tunnel: [w302 w303] -> w28
        tunnel: w23 -> [w301 _]
        frame False {
        }
        frame True {
          # "Write settings back to XML"
          n194 = Flatten To XML(anything=w303) -> (xml string=w305:string)
          n195 = call "Get Config File Path.vi"() -> ("XML File Path"=w306:path)  [unwired: 10 in, 1 out]
          n196 = call-poly <vilib>:"Write to XML File.vi"("XML Input"=w305, "XML File Path"=w306) -> ("error out"=w304:errorcluster)  [unwired: 7 in, 2 out]
        }
      }
    }
    frame Error {
    }
  }
  "UI Refresh Needed?" <- w14
  "error out" <- w15
  "Cancelled?" <- w13
  "TCU Module Config Out" <- w9
